vi "Find Test and Suite Index.vi"(8 "error in (no error)":errorcluster, 11 "Linker.Read Info From File":T2(array[cluster])) -> (0 "error out":errorcluster, 2 "Define Test index":i32, 3 "Define Test Suite index":i32)   [LabVIEW 2013, in "Caraya.lvlib" / "Test Runner.Folder.lvclass"]
uses:
  Test Runner.Folder.lvclass
  <vilib>/Utility/lvfile.llb/LVFileType.ctl
  Test/Define Test.vi
  Test Suite/Define Test Suite.vi
  Test/Test.lvclass
  Test Suite/Test Suite.lvclass
  <vilib>/Utility/lvfile.llb/NI_FileType.lvlib
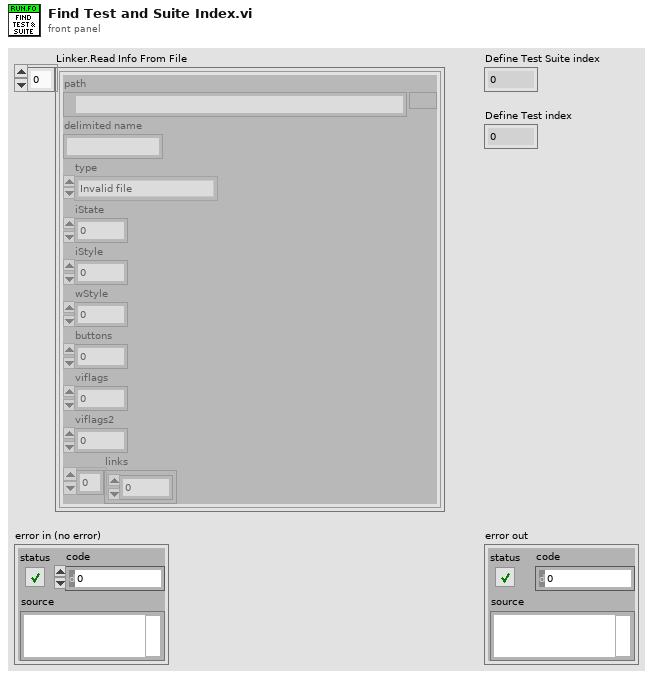
[diagram p1: front panel]
types:
  T1 = typedef "NI_FileType.lvlib/LVFileType.ctl" = enum32{"Invalid file", "Unknown type", "Instrument", "Control", "Polymorphic VI", "Project", "Library", "LVClass", "XControl", "XNode", "Shared library", ".NET assembly", "ActiveX interface", "CIN", "Run-time menu", "Palette menu", "Help file", "LLB", "XNode Edit Dependency", "Class Private Data Control", "Statechart", "MathScript .m file", "Ladder Diagram", "LVLibp", "XNode Build Dependency"}
  T2 = cluster{"path":path, "delimited name":string, "type":T1, "iState":u32, "iStyle":u16, "wStyle":u16, "buttons":u16, "viflags":u32, "viflags2":u32, "links":u32[]}[]
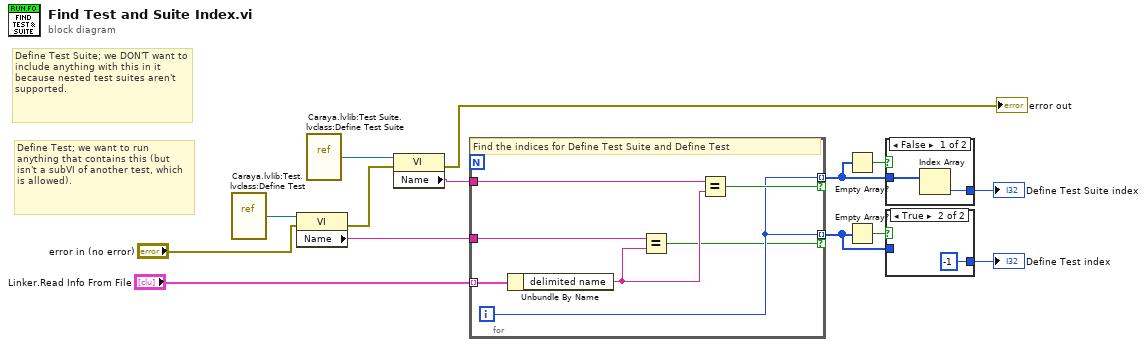
[diagram p0: block diagram]
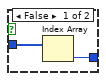
[diagram p2: hidden frame]
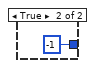
[diagram p3: hidden frame]
diagram:
  # "Define Test; we want to run anything that contains this (but isn't a subVI of another test, which is allowed)."
  # "Define Test Suite; we DON'T want to include anything with this in it because nested test suites aren't supported."
  n1 = vi-ref "Caraya.lvlib:Test.lvclass:Define Test.vi"() -> (w6:refnum<vi>)
  n2 = property class="VI"(reference=w6, error in="error in (no error)") -> (error out=w9:errorcluster, "Name"=w11:string)  [unwired: 1 out]
  n3 = vi-ref "Caraya.lvlib:Test Suite.lvclass:Define Test Suite.vi"() -> (w8:refnum<vi>)
  n4 = property class="VI"(reference=w8, error in=w9) -> (error out=→"error out":errorcluster, "Name"=w10:string)  [unwired: 1 out]
  n5 = for {
    tunnel: "Linker.Read Info From File" -> [w21] mode=indexing
    tunnel: w10 -> [w19]
    tunnel: w11 -> [w20]
    tunnel: [w16] -> w5 mode=indexing if=w17
    tunnel: [w16] -> w2 mode=indexing if=w15
    i -> [w16]
    # "Find the indices for Define Test Suite and Define Test"
    n6 = Unbundle By Name(w21) -> ("delimited name"=w18:string)
    n7 = Equal?(x=w20, y=w18) -> (x = y?=w15:bool)
    n8 = Equal?(x=w19, y=w18) -> (x = y?=w17:bool)
  }
  n9 = Empty Array?(array=w5) -> (empty?=w4:bool)
  n10 = Empty Array?(array=w2) -> (empty?=w3:bool)
  n11 = case shown="False" w4 {
    tunnel: [w23 -1] -> w13
    tunnel: w5 -> [w22 _]
    frame False {
      n12 = Index Array(array=w22) -> (element=w23:i32)  [unwired: 1 in]
    }
    frame True {
    }
  }
  "Define Test Suite index" <- w13
  n13 = case shown="True" w3 {
    tunnel: [w26 -1] -> w1
    tunnel: w2 -> [w25 _]
    frame False {
      n14 = Index Array(array=w25) -> (element=w26:i32)  [unwired: 1 in]
    }
    frame True {
    }
  }
  "Define Test index" <- w1
